vi "Get Instrument VI Paths.vi"(8 "error in (no error)":errorcluster) -> (0 "error out":errorcluster, 3 "Instr VI Paths[]":path[](array[path]))   [LabVIEW 2021, in "Migrator Reusables.lvlib"]
uses:
  Migrator Reusables.lvlib
  controls/Dictionary States.ctl
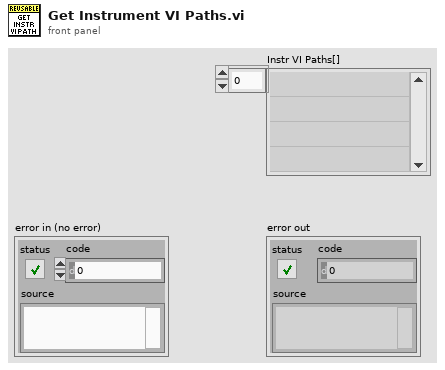
[diagram p1: front panel]
types:
  T1 = typedef "Migrator Reusables.lvlib/Dictionary States.ctl" = enum16{"Set", "Get", "Delete", "Delete All"}
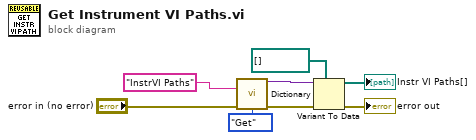
[diagram p0: block diagram]
diagram:
  n1 = call "Dictionary.vi"("Key"="InstrVI Paths", "error in (no error)"="error in (no error)", "Dict States"=Dictionary_States."Get") -> ("Variant_Out"=w4:variant, "error out"=w5:errorcluster)  [unwired: 11 in]
  n2 = Variant To Data(error in=w5, type=path[] [], Variant=w4) -> (data=→"Instr VI Paths[]":path[], error out=→"error out":errorcluster)
